vi "On Compile - Get Asynchronous Channels Status Block Refs.vi"(8 "error in":errorcluster, 11 "custom device ref":T1 format="%.0x") -> (0 "error out":errorcluster, 3 "Async Status Channels Refs":T2 {"VS Refs" format="%.0x"})   [LabVIEW 2020, in "AIM ARINC 429 System Explorer.lvlib" / "Implementation.lvlib"]
uses:
  Implementation.lvlib
  <vilib>/NI VeriStand/Custom Device API/Custom Device Item Ref.ctl
  <vilib>/NI VeriStand/Custom Device API/Custom Device API.lvlib
  Scripting/AIM/Constants.vi
  Scripting/AIM/AIM ARINC 429 Scripting.lvlib
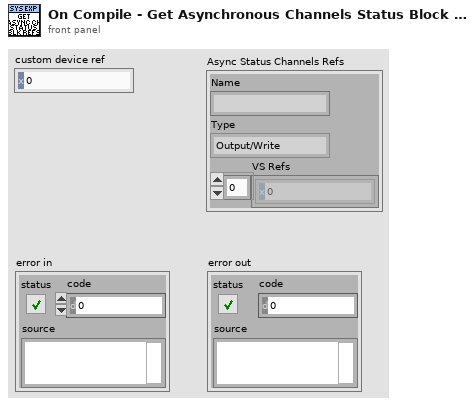
[diagram p1: front panel]
types:
  T1 = typedef "Custom Device API.lvlib/Custom Device Item Ref.ctl" = u64
  T2 = cluster{"Name":string, "Type":enum16{"Output/Write", "Input/Read", "Input/ReadWrite"}, "VS Refs":T1[]}
  T3 = enum16{"Output/Write", "Input/Read", "Input/ReadWrite"}
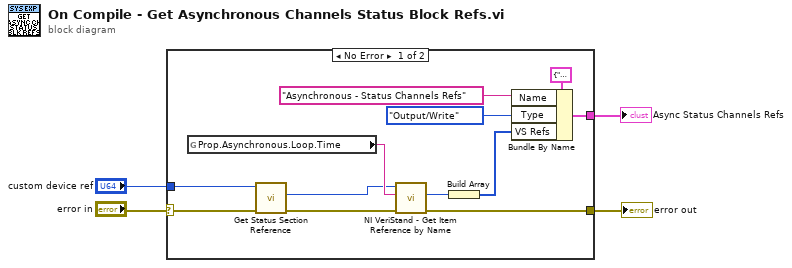
[diagram p0: block diagram]
diagram:
  n1 = case shown="No Error" "error in" {
    selector: "error in" -> [w7 w17]
    tunnel: "custom device ref" -> [w8 _]
    tunnel: [w10 w17] -> w2
    tunnel: [w13 _] -> w1
    frame No Error {
      n2 = global read "Constants.vi" "Prop.Asynchronous.Loop.Time"() -> (w9:string)
      n3 = call "Get Status Section Reference.vi"("error in"=w7, "Ballard ARINC 429 ref"=w8) -> ("error out"=w5:errorcluster, "status section reference"=w6:T1)  [unwired: 7 in, 1 out]
      n4 = call <vilib>:"NI VeriStand - Get Item Reference by Name.vi"("error in (no error)"=w5, "Item Name"=w9, "Parent Ref in"=w6) -> ("error out"=w10:errorcluster, "Item Ref"=w16:T1)  [unwired: 5 in, 2 out]
      n5 = Build Array(w16) -> (w12:T1[])
      n6 = Bundle By Name(cluster=T2 {"Name"="", "Type"=enum."Output/Write", "VS Refs"=[]} ("Group"), "Name"="Asynchronous - Status Channels Refs", "Type"=T3."Output/Write", "VS Refs"=w12) -> (w13:T2)
    }
    frame Error {
    }
  }
  "error out" <- w2
  "Async Status Channels Refs" <- w1
